vi "Novo_tempo_obs.vi"() -> (2 "TO horas":dbl, 3 "TO rad":dbl)   [LabVIEW 2018]
uses:
  Global_Telescopio.vi
panel:
  out "Numeric":i32
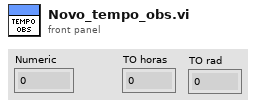
[diagram p1: front panel]
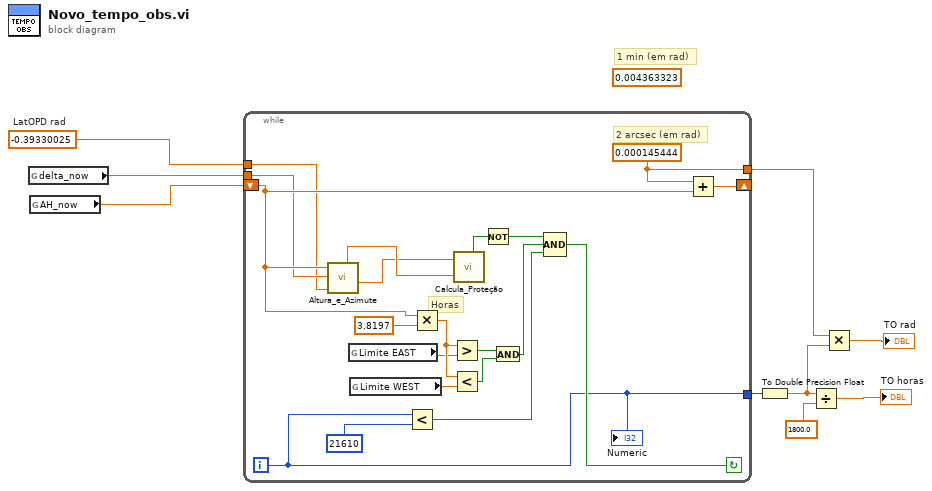
[diagram p0: block diagram]
diagram:
  w1 = -0.39330025  # LatOPD rad
  (unwired) 0.004363323
  # "1 min (em rad)"
  n1 = global read "Global_Telescopio.vi" "delta_now"() -> (w3:dbl)
  n2 = global read "Global_Telescopio.vi" "AH_now"() -> (w2:dbl)
  n3 = while {
    tunnel: w1 -> [w12]
    tunnel: w3 -> [w13]
    shift-right: [w19] -> _
    shift-left: w2 -> [w14]
    tunnel: [w17] -> w9
    tunnel: [w18] -> w6
    i -> [w17]
    stop <- w20 continue-if-true
    w18 = 0.000145444
    # "2 arcsec (em rad)"
    # "Horas"
    n4 = call "Altura_e_Azimute.vi"("LAT rad"=w12, "DEC rad"=w13, "AH rad"=w14) -> ("AZIMUTE rad"=w10:dbl, "ANG. ZENITAL rad"=w11:dbl)  [unwired: 4 out]
    n5 = global read "Global_Telescopio.vi" "Limite EAST"() -> (w23:dbl)
    n6 = global read "Global_Telescopio.vi" "Limite WEST"() -> (w24:dbl)
    n7 = Less?(x=w17, y=21610) -> (x < y?=w15:bool)
    n8 = Multiply(x=w14, y=3.8197) -> (x*y=w27:dbl)
    n9 = Greater?(x=w27, y=w23) -> (0:w26:bool)
    n10 = Less?(x=w27, y=w24) -> (x < y?=w22:bool)
    n11 = call "Calcula_Proteção.vi"("Zenital angle rad"=w11, "Azimute rad"=w10) -> ("Prot Zmax"=w29:bool)  [unwired: 4 out]
    n12 = Not(x=w29) -> (.not. x?=w25:bool)
    n13 = And(x=w26, y=w22) -> (x .and. y?=w21:bool)
    n14 = Compound Arithmetic op=AND(w25, w21, w15) -> (w20:bool)
    n15 = Add(x=w18, y=w14) -> (x+y=w19:dbl)
    "Numeric" <- w17
  }
  n16 = To Double Precision Float(number=w9) -> (double precision float=w5:dbl)
  n17 = Divide(x=w5, y=1800.0) -> (x/y=→"TO horas":dbl)
  n18 = Multiply(x=w6, y=w5) -> (x*y=→"TO rad":dbl)
